vi "Alpha sort 2D.vi"(1 "Column Number":i32=2, 2 "Input Array":string[][](array[string])) -> (0 "Sorted Array":string[][](array[string]))   [LabVIEW 2014]
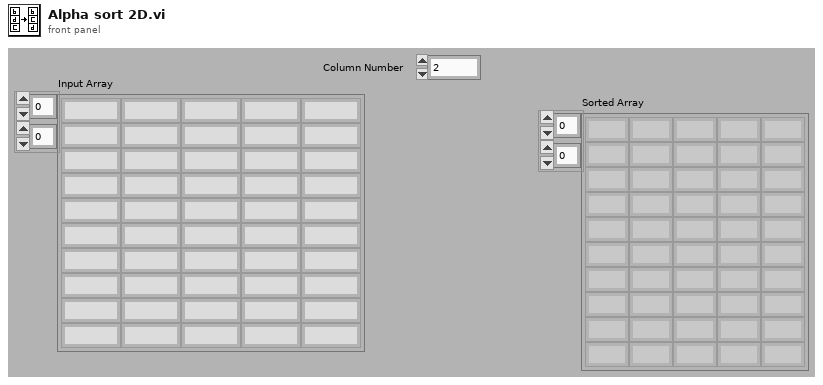
[diagram p1: front panel]
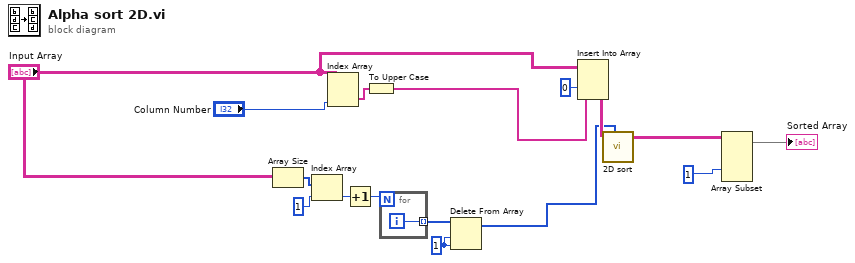
[diagram p0: block diagram]
diagram:
  w2 = 1 ("Index")
  n1 = Array Size(array="Input Array") -> (size(s)=w7:i32[])
  n2 = Index Array(array=w7, index=1 ("Array Index")) -> (element=w5:i32)
  n3 = Index Array(array="Input Array", index (col)="Column Number") -> (element=w14:string[])  [unwired: 1 in]
  n4 = Increment(x=w5) -> (x+1=w1:i32)
  n5 = To Upper Case(1:w14) -> (0:w11:string[])
  n6 = for {
    N: w1 -> [_]
    tunnel: [w17] -> w4 mode=indexing
    i -> [w17]
  }
  n7 = Delete From Array(array=w4, length=w2, index=w2) -> (array with subset deleted=w3:i32[])  [unwired: 1 out]
  n8 = Insert Into Array(array="Input Array", index (col)=0, new element=w11) -> (w16:string[][])  [unwired: 1 in]
  n9 = call "2D sort.vi"("Column Sort Order"=w3, "Array In"=w16) -> ("Array Out"=w10:string[][])  [unwired: 9 in]
  n10 = Array Subset(array=w10, index (col)=1 ("Array Index")) -> (→"Sorted Array":string[][])  [unwired: 3 in]
